vi "Lissajous_Patterns.vi"() -> ()   [LabVIEW 2022 SP3]
panel:
  in  "Resolution B":dbl
  in  "Resolution A":dbl
  in  "# of Harmonics":i32=11
  in  "Sample Rate A":i32=16384
  in  "Sample Rate B":i32=16384
  in  "Initial Phase B (0-2pi)":dbl[](array[slide]) scale=0.0..6.28
  in  "Rate of phase change":dbl[](array[slide]) scale=0.0..0.5
  in  "stop":bool
  in  "Amplitude A (1/x)":dbl[][](array[numeric]) min=0.0 max=50.0
  in  "*Adjustable* Phase A (0-2pi)":dbl[](array[slide]) scale=0.0..6.28
  in  "Amplitude B (1/x)":dbl[][](array[numeric]) min=0.0 max=50.0
  out "XY Graph":cluster{dbl[], dbl[]}(graph)
  # "Notes: \n\nThe number of harmonics can be increased. If you change the number of harmonics, ensure that the number of options available for the amp/phase/rate of change matches.\n\nThe sample rate of A and B should usually match.\n\nMore info on Lissajous Patterns can be found on wikipedia https://en.wikipedia.org/wiki/Lissajous_curve\n\nIn general, the patterns help us visualize ratios between frequencies A and B along with their phase offset."
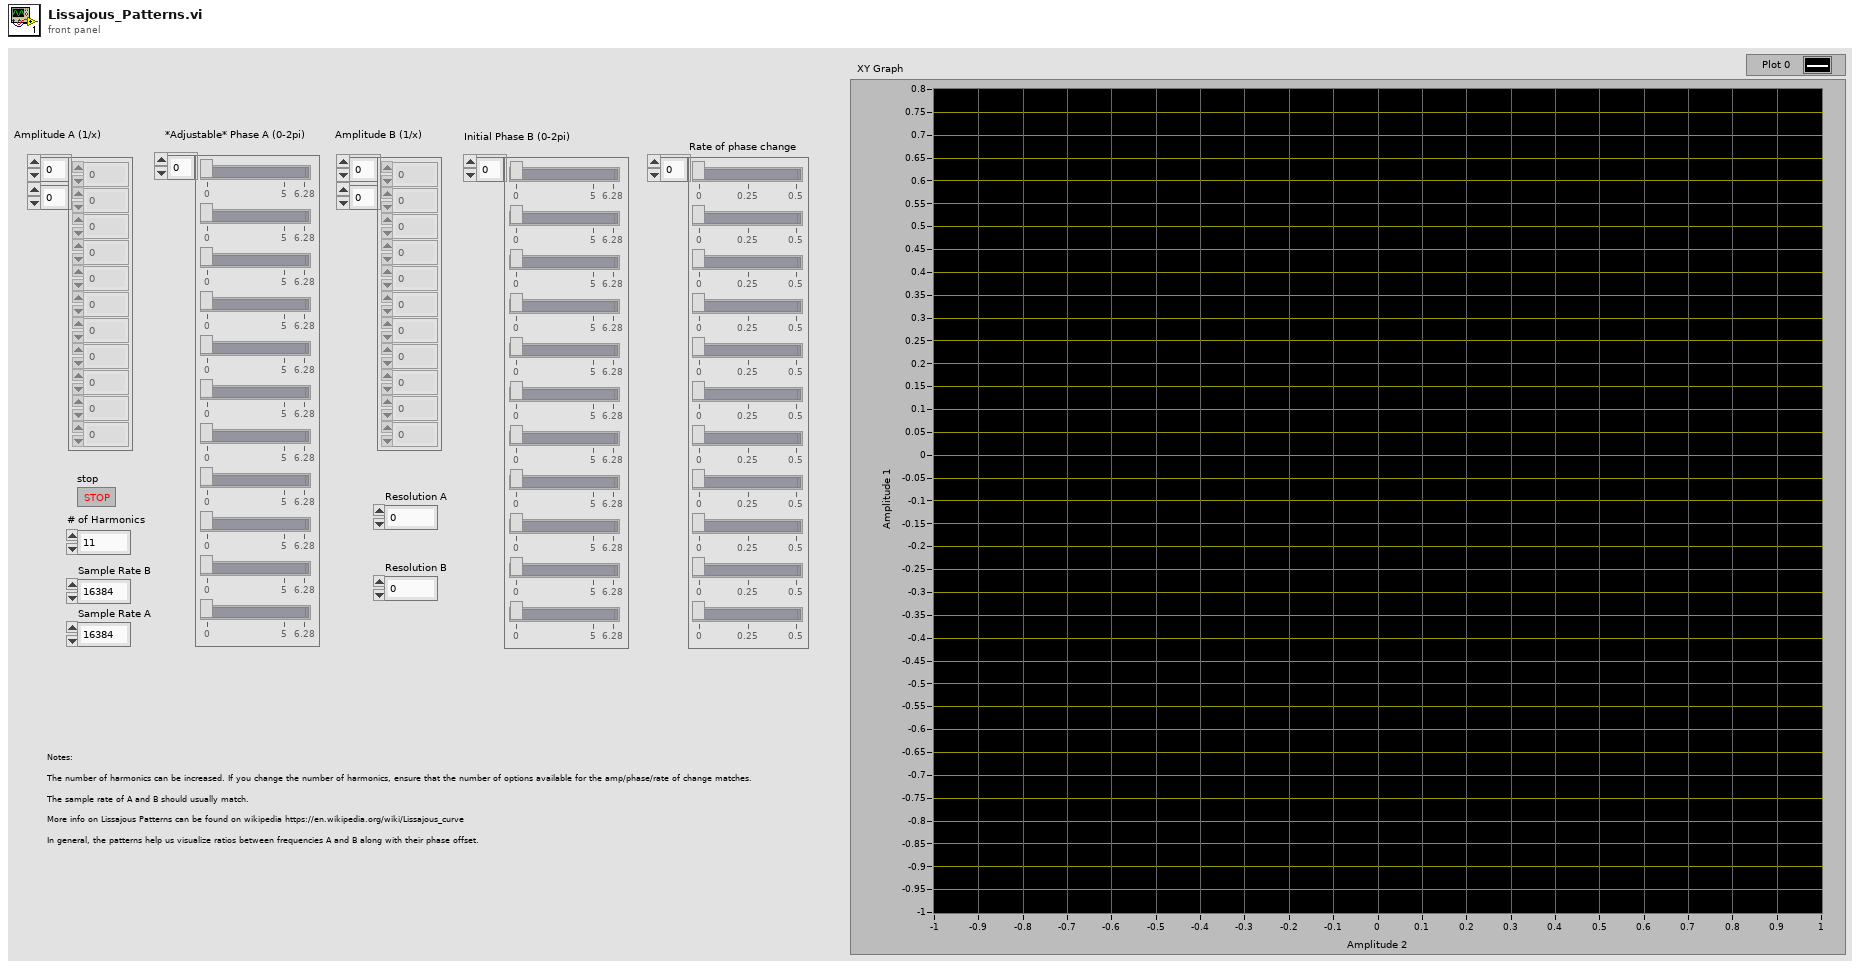
[diagram p1: front panel]
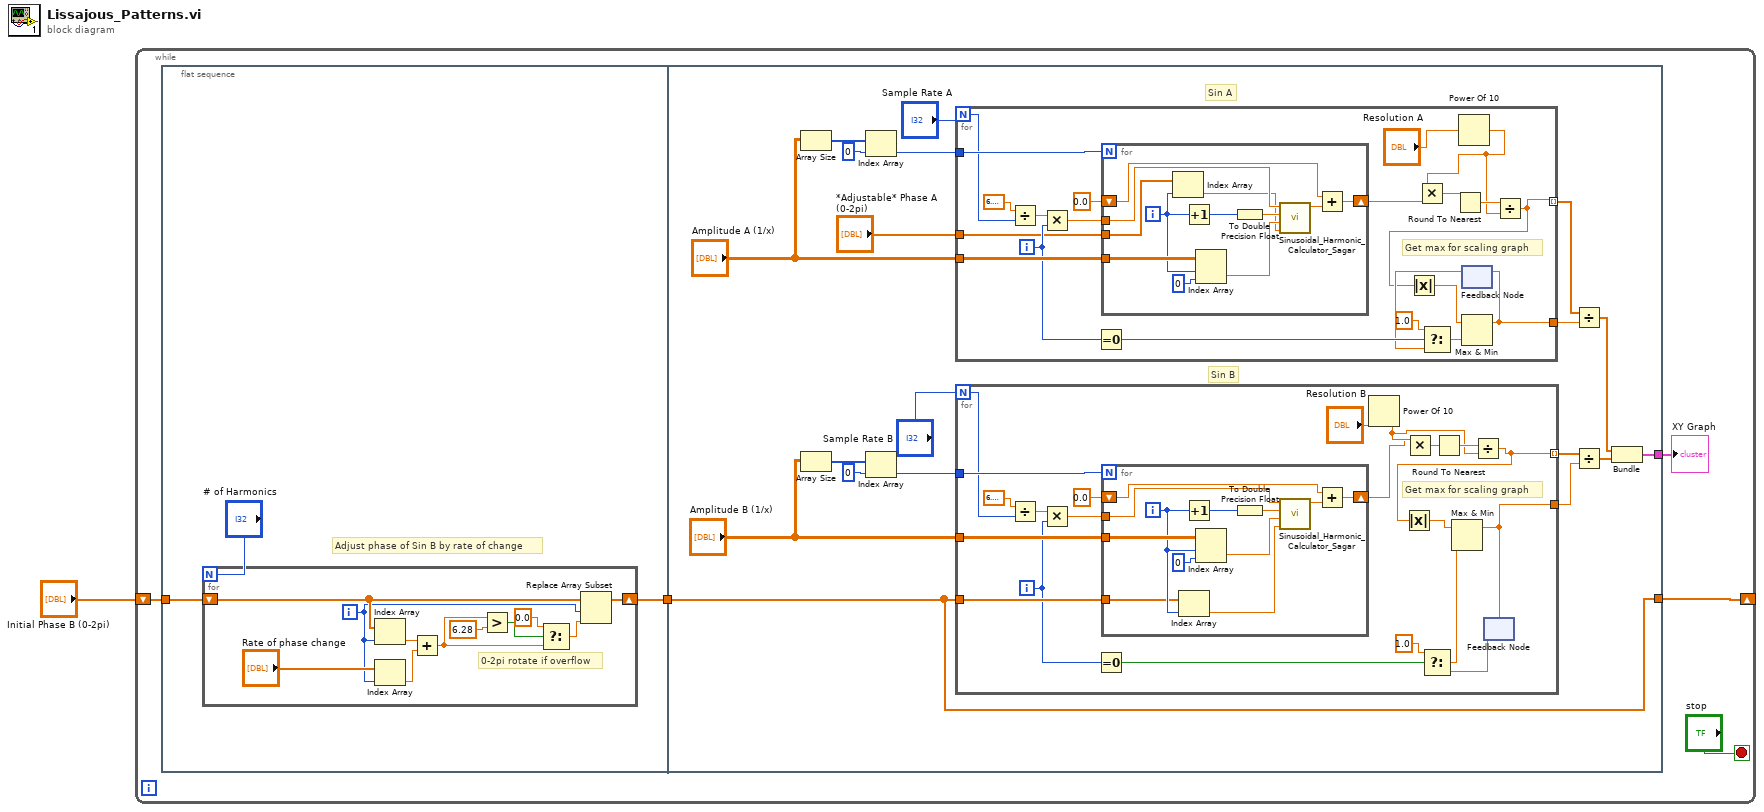
[diagram p0: block diagram]
diagram:
  n1 = while {
    shift-right: [w4] -> _
    shift-left: "Initial Phase B (0-2pi)" -> [w2]
    stop <- "stop" stop-if-true
    n2 = flat-sequence {
      tunnel: [w9] -> w5
      tunnel: w2 -> [w8]
      tunnel: [w25] -> w3
      tunnel: w5 -> [w24]
      tunnel: [w24] -> w4
      frame #0 {
        # "Adjust phase of Sin B by rate of change"
        n3 = for {
          N: "# of Harmonics" -> [_]
          shift-right: [w12] -> w9
          shift-left: w8 -> [w13]
          i -> [w11]
          # "0-2pi rotate if overflow"
          n4 = Index Array(array=w13, index=w11) -> (element=w14:dbl)
          n5 = Index Array(array="Rate of phase change", index=w11) -> (element=w15:dbl)
          n6 = Add(x=w14, y=w15) -> (x+y=w17:dbl)
          n7 = Greater?(x=w17, y=6.28) -> (0:w19:bool)
          n8 = Select(t=0.0, s=w19, f=w17) -> (s? t:f=w10:dbl)
          n9 = Replace Array Subset(array=w13, new element=w10, index=w11) -> (w12:dbl[])
        }
      }
      frame #1 {
        # "Sin B"
        # "Sin A"
        n10 = Array Size(array="Amplitude A (1/x)") -> (size(s)=w28:i32[])
        n11 = Array Size(array="Amplitude B (1/x)") -> (size(s)=w33:i32[])
        n12 = Index Array(array=w28, index=0) -> (element=w30:i32)
        n13 = Index Array(array=w33, index=0) -> (element=w35:i32)
        n14 = for {
          N: "Sample Rate A" -> [w86]
          tunnel: w30 -> [w91]
          tunnel: "Amplitude A (1/x)" -> [w88]
          tunnel: [w73] -> w31 mode=indexing
          tunnel: [w80] -> w32
          tunnel: "*Adjustable* Phase A (0-2pi)" -> [w79]
          i -> [w82]
          # "Get max for scaling graph"
          n15 = Divide(x=6.283185307179586, y=w86) -> (x/y=w92:dbl)
          n16 = Multiply(x=w92, y=w82) -> (x*y=w90:dbl)
          n17 = Equal To 0?(x=w82) -> (x = 0?=w85:bool)
          n18 = for {
            N: w91 -> [_]
            tunnel: w90 -> [w105]
            shift-right: [w103] -> w74
            shift-left: 0.0 -> [w104]
            tunnel: w88 -> [w101]
            tunnel: w79 -> [w95]
            i -> [w96]
            n19 = Index Array(array=w95, index=w96) -> (element=w94:dbl)
            n20 = Increment(x=w96) -> (x+1=w99:i32)
            n21 = Index Array(array=w101, index (row)=w96, index (col)=0 ("disabled index (col)")) -> (element=w97:dbl)
            n22 = To Double Precision Float(number=w99) -> (double precision float=w98:dbl)
            n23 = call "Sinusoidal_Harmonic_Calculator_Sagar.vi"("Phase"=w94, "Amplitude (1/x)"=w97, "Harmonic"=w98, "Numeric in"=w105) -> ("Numeric out"=w102:dbl)  [unwired: 7 in]
            n24 = Add(x=w104, y=w102) -> (x+y=w103:dbl)
          }
          n25 = Power Of 10(x="Resolution A") -> (10^x=w75:dbl)
          n26 = Multiply(x=w75, y=w74) -> (x*y=w78:dbl)
          n27 = Round To Nearest(number=w78) -> (nearest integer value=w77:dbl)
          n28 = feedback #1() -> (w84:dbl)  [unwired: 1 in]
          n29 = Select(t=1.0, s=w85, f=w84) -> (s? t:f=w81:dbl)
          n30 = Divide(x=w77, y=w75) -> (x/y=w73:dbl)
          n31 = Absolute Value(x=w73) -> (abs(x)=w87:dbl)
          n32 = Max & Min(x=w87, y=w81) -> (max(x,y)=w80:dbl)  [unwired: 1 out]
          n33 = feedback-in #1(w80) -> ()
        }
        n34 = for {
          N: "Sample Rate B" -> [w52]
          tunnel: w35 -> [w58]
          tunnel: "Amplitude B (1/x)" -> [w55]
          tunnel: [w40] -> w36 mode=indexing
          tunnel: w24 -> [w54]
          tunnel: [w46] -> w37
          i -> [w48]
          # "Get max for scaling graph"
          n35 = Divide(x=6.283185307179586, y=w52) -> (x/y=w59:dbl)
          n36 = Multiply(x=w59, y=w48) -> (x*y=w57:dbl)
          n37 = Equal To 0?(x=w48) -> (x = 0?=w51:bool)
          n38 = for {
            N: w58 -> [_]
            tunnel: w57 -> [w72]
            shift-right: [w70] -> w41
            shift-left: 0.0 -> [w71]
            tunnel: w55 -> [w68]
            tunnel: w54 -> [w62]
            i -> [w63]
            n39 = Index Array(array=w62, index=w63) -> (element=w61:dbl)
            n40 = Increment(x=w63) -> (x+1=w66:i32)
            n41 = Index Array(array=w68, index (row)=w63, index (col)=0 ("disabled index (col)")) -> (element=w64:dbl)
            n42 = To Double Precision Float(number=w66) -> (double precision float=w65:dbl)
            n43 = call "Sinusoidal_Harmonic_Calculator_Sagar.vi"("Phase"=w61, "Amplitude (1/x)"=w64, "Harmonic"=w65, "Numeric in"=w72) -> ("Numeric out"=w69:dbl)  [unwired: 7 in]
            n44 = Add(x=w71, y=w69) -> (x+y=w70:dbl)
          }
          n45 = Power Of 10(x="Resolution B") -> (10^x=w42:dbl)
          n46 = Multiply(x=w41, y=w42) -> (x*y=w44:dbl)
          n47 = Round To Nearest(number=w44) -> (nearest integer value=w43:dbl)
          n48 = Divide(x=w43, y=w42) -> (x/y=w40:dbl)
          n49 = Absolute Value(x=w40) -> (abs(x)=w53:dbl)
          n50 = feedback #2() -> (w50:dbl)  [unwired: 1 in]
          n51 = Select(t=1.0, s=w51, f=w50) -> (s? t:f=w47:dbl)
          n52 = Max & Min(x=w53, y=w47) -> (max(x,y)=w46:dbl)  [unwired: 1 out]
          n53 = feedback-in #2(w46) -> ()
        }
        n54 = Divide(x=w31, y=w32) -> (x/y=w39:dbl[])
        n55 = Divide(x=w36, y=w37) -> (x/y=w38:dbl[])
        n56 = Bundle(w39, w38) -> (w25:cluster{dbl[], dbl[]})  [unwired: 1 in]
      }
    }
    "XY Graph" <- w3
  }
